vi "Add Custom Symbol.vi"(8 "error in":errorcluster, 9 "Symbol ID":string, 10 "Symbol File Path":path, 11 "Tree Map":refnum<class "Project Tree Map.lvclass">) -> (0 "error out":errorcluster, 3 "Tree Map":refnum<class "Project Tree Map.lvclass">)   [LabVIEW 2020, in "VI Properties Editor.lvlib" / "Project Tree Map.lvclass"]
doc: "Adds a custom symbol to the tree map."
uses:
  Project Tree Map.lvclass
  <vilib>/picture/picture.llb/imagedata.ctl
  Project Tree Map.lvclass/Project Tree Map.ctl
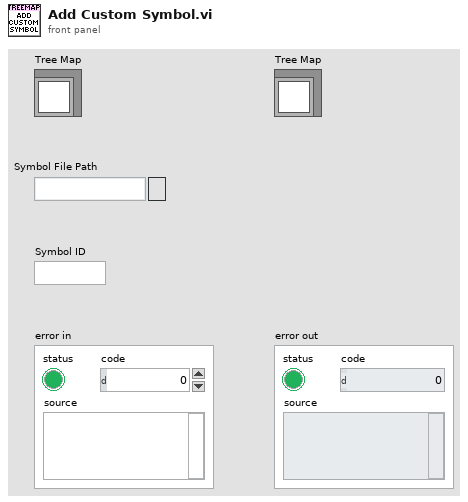
[diagram p1: front panel]
types:
  T1 = typedef "imagedata.ctl" = cluster{"image type":i32, "image depth":i32, "image":u8[], "mask":u8[], "colors":u32[], "Rectangle":cluster{"left":i16, "top":i16, "right":i16, "bottom":i16}}
  T2 = map{string, cluster{"index":i32, "image data":T1}}
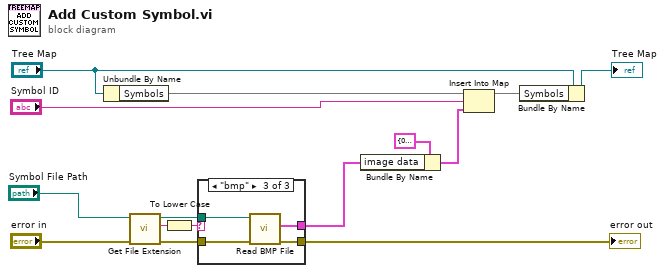
[diagram p0: block diagram]
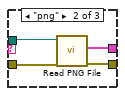
[diagram p3: hidden frame]
diagram:
  n1 = Unbundle By Name("Tree Map") -> ("Symbols"=w7:T2)
  n2 = call <vilib>:"Get File Extension.vi"("error in (no error)"="error in", "file"="Symbol File Path") -> ("error out"=w12:errorcluster, "lowercase file extension"=w14:string, "dup file"=w13:path)  [unwired: 5 in, 2 out]
  n3 = To Lower Case(string=w14) -> (all lower case string=w9:string)
  n4 = case shown="\"bmp\"" w9 {
    tunnel: w13 -> [_ w17 w24]
    tunnel: w12 -> [w16 w20 w23]
    tunnel: [_ w18 w22] -> w4
    tunnel: [w16 w19 w21] -> w10
    frame Default {
    }
    frame "png" {
      n5 = call <vilib>:"Read PNG File.vi"("error in (no error)"=w20, "path to PNG file"=w17) -> ("error out"=w19:errorcluster, "image data"=w18:T1)  [unwired: 7 in, 1 out]
    }
    frame "bmp" {
      n6 = call <vilib>:"Read BMP File.vi"("error in (no error)"=w23, "path to BMP file"=w24) -> ("error out"=w21:errorcluster, "image data"=w22:T1)  [unwired: 7 in, 1 out]
    }
  }
  "error out" <- w10
  n7 = Bundle By Name(cluster=cluster{"index":i32, "image data":T1} {"index"=0, "image data"={"image type"=0, "image depth"=0, "image"=[], "mask"=[], "colors"=[], "Rectangle"={"left"=0, "top"=0, "right"=0, "bottom"=0}}} ("value"), "image data"=w4) -> (w1:cluster{"index":i32, "image data":T1})
  n8 = Insert Into Map(map in=w7, key="Symbol ID", value=w1) -> (map out=w2:T2)  [unwired: 2 out]
  n9 = Bundle By Name(cluster="Tree Map", "Symbols"=w2) -> (→"Tree Map":refnum<class "Project Tree Map.lvclass">)
